vi "Dashboard exit vi.vi"(8 "error in (no error)":errorcluster, 10 "Exit in":bool, 11 "Enum":enum16{"Write", "Read"}(ring)) -> (0 "error out":errorcluster, 3 "Exit Out":bool)   [LabVIEW 2017]
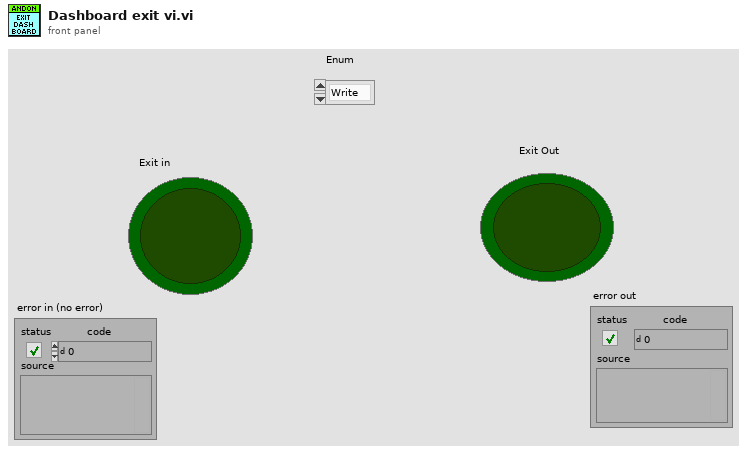
[diagram p1: front panel]
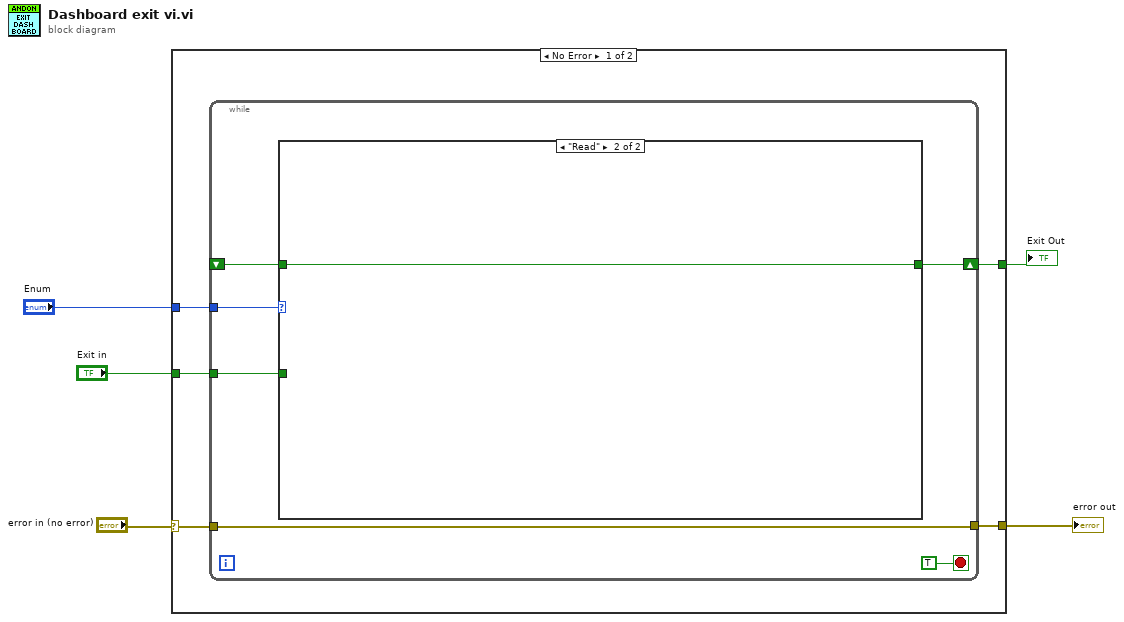
[diagram p0: block diagram]
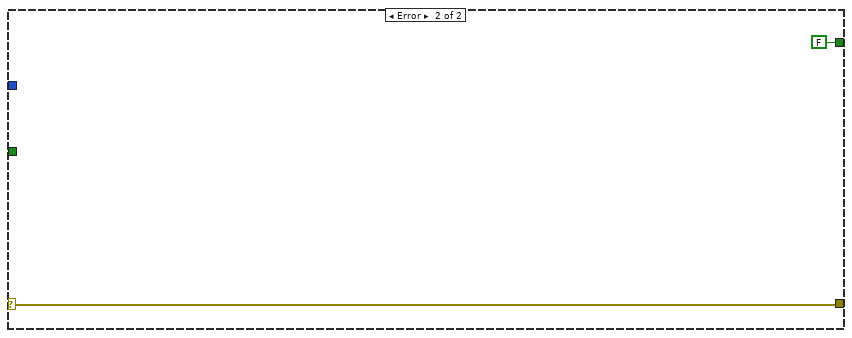
[diagram p3: hidden frame]
diagram:
  n1 = case shown="No Error" "error in (no error)" {
    selector: "error in (no error)" -> [w9 w20]
    tunnel: [w10 w20] -> w4
    tunnel: "Enum" -> [w8 _]
    tunnel: [w7 FALSE ("Exit in")] -> w1
    tunnel: "Exit in" -> [w6 _]
    frame No Error {
      n2 = while {
        tunnel: [w15] -> w10
        tunnel: w9 -> [w15]
        tunnel: w8 -> [w14]
        tunnel: w6 -> [w12]
        shift-right: [w13] -> w7
        shift-left: _ -> [w11]
        stop <- TRUE stop-if-true
        n3 = case shown="\"Read\"" w14 {
          tunnel: [w17 w18] -> w13
          tunnel: w12 -> [w17 _]
          tunnel: w11 -> [_ w18]
          frame "Write", Default {
          }
          frame "Read" {
          }
        }
      }
    }
    frame Error {
    }
  }
  "Exit Out" <- w1
  "error out" <- w4
